vi "test_UMB_vis.vi"() -> ()   [LabVIEW 2020]
uses:
  BlockMessage/ubm_value_type.ctl
  BlockMessage/UdpBlockMessage.lvlib
panel:
  in  "# of messages":i32
  out "Message Block Array":u32[](array[numeric])
  out "Udp Block Message Map":map{i32, T1}(c390)
  in  "Data in":u8[](array[numeric])
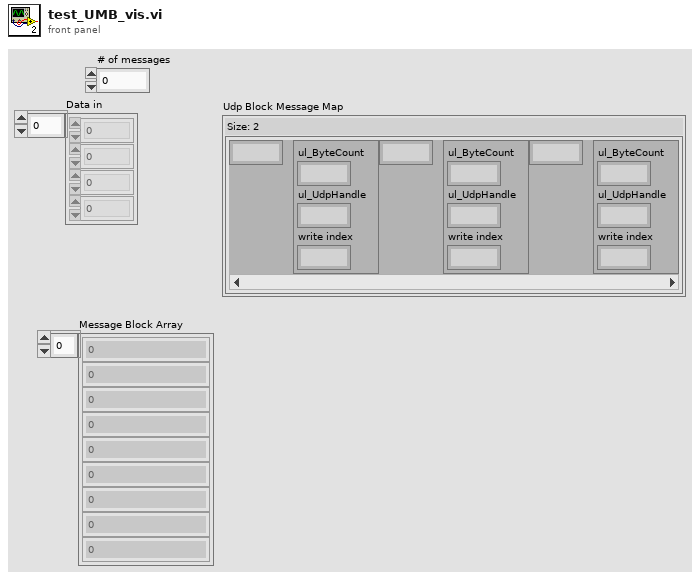
[diagram p1: front panel]
types:
  T1 = typedef "UdpBlockMessage.lvlib/ubm_value_type.ctl" = cluster{"ul_ByteCount":u32, "ul_UdpHandle":u32, "write index":u32}
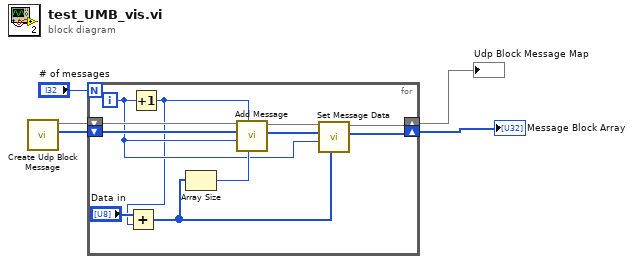
[diagram p0: block diagram]
diagram:
  n1 = call "Create Udp Block Message.vi"() -> ("Message Block Array"=w4:u32[], "Udp Block Message Map"=w5:map{i32, T1})  [unwired: 9 in, 1 out]
  n2 = for {
    N: "# of messages" -> [_]
    shift-right: [w11] -> w3
    shift-left: w5 -> [w16]
    shift-right: [w12] -> w2
    shift-left: w4 -> [w14]
    i -> [w8]
    n3 = Increment(x=w8) -> (x+1=w6:i32)
    n4 = Add(x="Data in", y=w6) -> (x+y=w7:i32[])
    n5 = Array Size(array=w7) -> (size(s)=w10:i32)
    n6 = call "Add Message.vi"("ul_ByteCount"=w10, "ul_UdpHandle"=w6, "index"=w8, "Message Block Array in"=w14, "Udp Block Message Map in"=w16) -> ("Message Block Array out"=w13:u32[], "Udp Block Message Map out"=w15:map{i32, T1})  [unwired: 4 in, 1 out]
    n7 = call "Set Message Data.vi"("Data in"=w7, "index"=w8, "Message Block Array in"=w13, "Udp Block Message Map in"=w15) -> ("Message Block Array out"=w12:u32[], "Udp Block Message Map out"=w11:map{i32, T1})  [unwired: 5 in, 1 out]
  }
  "Udp Block Message Map" <- w3
  "Message Block Array" <- w2
